vi "Stop Core.vi"(10 "final error code":i32, 11 "Manager in":refnum<class "Manager.lvclass">) -> (3 "Manager out":refnum<class "Manager.lvclass">)   [LabVIEW 2012, in "Manager.lvlib" / "Manager.lvclass"]
uses:
  Manager.lvclass
  <vilib>/ActorFramework/Actor/Actor.lvclass
  Manager.lvclass/Manager.ctl
  <vilib>/ActorFramework/Stop Msg/Stop Msg.lvclass/Stop Msg.ctl
  <vilib>/ActorFramework/Message Enqueuer/Message Enqueuer.lvclass/Message Enqueuer.ctl
  Read Control Systems.vi
  <vilib>/ActorFramework/Stop Msg/Send Emergency Stop.vi
  <vilib>/ActorFramework/Stop Msg/Send Normal Stop.vi
  <vilib>/ActorFramework/Message Enqueuer/Enqueue Critical.vi
  <vilib>/ActorFramework/Message Enqueuer/Enqueue.vi
  <vilib>/ActorFramework/Message Priority Queue/Priority Enqueue.vi
  <vilib>/ActorFramework/Stop Msg/Stop Msg.lvclass
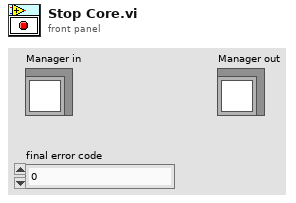
[diagram p1: front panel]
types:
  T1 = cluster{"Bioreactor Queue":refnum<class "Message Enqueuer.lvclass">, "Time Protocol Queue":refnum<class "Message Enqueuer.lvclass">, "Python Protocol Queue":refnum<class "Message Enqueuer.lvclass">, "Name":string}[]
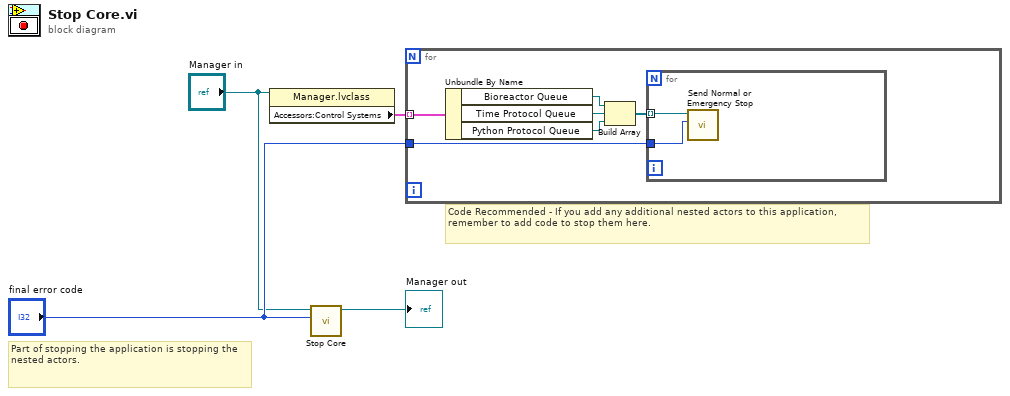
[diagram p0: block diagram]
diagram:
  # "Code Recommended - If you add any additional nested actors to this application, remember to add code to stop them here."
  # "Part of stopping the application is stopping the nested actors."
  n1 = property class="Manager.lvclass"(reference="Manager in") -> ("Accessors:Control Systems"=w1:T1)  [unwired: 1 in, 2 out]
  n2 = call-parent "Stop Core.vi"("final error code"="final error code", "Actor in"="Manager in") -> ("Actor out"=→"Manager out":refnum<class "Manager.lvclass">)  [unwired: 9 in]
  n3 = for {
    tunnel: "final error code" -> [w5]
    tunnel: w1 -> [w10] mode=indexing
    n4 = Unbundle By Name(w10) -> ("Bioreactor Queue"=w9:refnum<class "Message Enqueuer.lvclass">, "Time Protocol Queue"=w8:refnum<class "Message Enqueuer.lvclass">, "Python Protocol Queue"=w7:refnum<class "Message Enqueuer.lvclass">)
    n5 = Build Array(w9, w8, w7) -> (w6:refnum<class "Message Enqueuer.lvclass">[])
    n6 = for {
      tunnel: w6 -> [w12] mode=indexing
      tunnel: w5 -> [w11]
      n7 = call <vilib>:"Send Normal or Emergency Stop.vi"("final error code"=w11, "Message Enqueuer"=w12) -> ()  [unwired: 9 in, 1 out]
    }
  }
